vi "GasflaschenListe_SpalteAblaufdatum_einfaerben.vi"(11 "MehrspaltigesListenfeld (Eingang)":refnum<vi>) -> ()   [LabVIEW 2020, in "System Einstellungen V2.lvlib"]
uses:
  System Einstellungen V2.lvlib
  <vilib>/Utility/miscctls.llb/LVRowAndColumnTypeDef.ctl
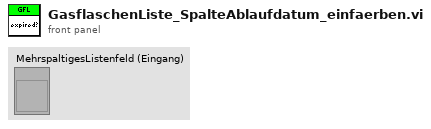
[diagram p1: front panel]
types:
  T1 = typedef "LVRowAndColumnTypeDef.ctl" = cluster{"Row":i32, "Column":i32}
  T2 = typedef "System Einstellungen V2.lvlib/Gasflasche gesamt.ctl" = cluster{"Gasflasche":T3, "Trägergas":T4, "Komponenten":T5[]}
  T3 = typedef "System Einstellungen V2.lvlib/Gasflasche.ctl" = cluster{"Gasname für die Auswahl":string, "Chargennummer":string, "Ablaufdatum":timestamp}
  T4 = typedef "System Einstellungen V2.lvlib/Traegergas.ctl" = string
  T5 = typedef "System Einstellungen V2.lvlib/Gasflaschenkomponente.ctl" = cluster{"Gasauswahl":string, "Konzentration IST":dbl, "Einheit":string, "Genauigkeit":dbl}
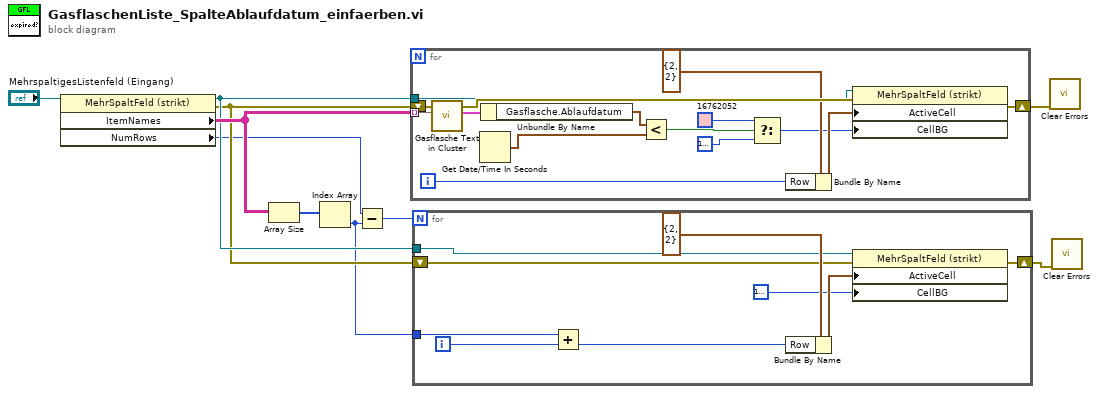
[diagram p0: block diagram]
diagram:
  n1 = property on="Eigenschaftsknoten" class="MehrSpaltFeld (strikt)"(reference="MehrspaltigesListenfeld (Eingang)") -> (reference out=w6:refnum<vi>, error out=w5:errorcluster, "ItemNames"=w8:string[][], "NumRows"=w3:u32)  [unwired: 1 in]
  n2 = Array Size(array=w8) -> (size(s)=w7:i32[])
  n3 = Index Array(array=w7) -> (element=w1:i32)  [unwired: 1 in]
  n4 = Subtract(x=w3, y=w1) -> (x-y=w2:u32)
  n5 = for {
    tunnel: w8 -> [w24] mode=indexing
    shift-right: [w20] -> w10
    shift-left: w5 -> [w21]
    tunnel: w6 -> [w11]
    i -> [w22]
    n6 = call "Gasflasche Text in Cluster.vi"("Gasflasche Text Array"=w24) -> ("Gasflasche"=w23:T2)  [unwired: 10 in]
    n7 = Get Date/Time In Seconds() -> (seconds since 1Jan1904=w18:timestamp)
    n8 = Unbundle By Name(w23) -> ("Gasflasche.Ablaufdatum"=w19:timestamp)
    n9 = Less?(x=w19, y=w18) -> (x < y?=w14:bool)
    n10 = Select(t=u32 16762052, s=w14, f=u32 16777216) -> (s? t:f=w13:u32)
    n11 = Bundle By Name(cluster=T1 {"Row"=2, "Column"=2} ("Aktive Zelle:Aktive Zelle"), "Row"=w22) -> (w16:T1)
    n12 = property on="Eigenschaftsknoten" class="MehrSpaltFeld (strikt)"(reference=w11, error in=w21, "ActiveCell"=w16, "CellBG"=w13) -> (error out=w20:errorcluster)  [unwired: 1 out]
  }
  n13 = for {
    N: w2 -> [_]
    tunnel: w6 -> [w29]
    shift-right: [w27] -> w4
    shift-left: w5 -> [w28]
    tunnel: w1 -> [w25]
    i -> [w30]
    n14 = Add(x=w25, y=w30) -> (x+y=w26:i32)
    n15 = Bundle By Name(cluster=T1 {"Row"=2, "Column"=2} ("Aktive Zelle:Aktive Zelle"), "Row"=w26) -> (w32:T1)
    n16 = property on="Eigenschaftsknoten" class="MehrSpaltFeld (strikt)"(reference=w29, error in=w28, "ActiveCell"=w32, "CellBG"=u32 16777216) -> (error out=w27:errorcluster)  [unwired: 1 out]
  }
  n17 = call <vilib>:"Clear Errors.vi"("error in (no error)"=w10) -> ()  [unwired: 5 in, 2 out]
  n18 = call <vilib>:"Clear Errors.vi"("error in (no error)"=w4) -> ()  [unwired: 5 in, 2 out]
